vi "Set CSR Mode.vi"(8 "error in (no error)":errorcluster, 10 "Bandpass resolution (per grating line)":enum16{"3600", "1800", "900", "450"}(ring), 11 "VISA resource name":refnum<visa-resource-name>) -> (0 "error out":errorcluster, 2 "Bandpass Value":dbl[unit] min=0.0 max=0.016777215000000012 step=1.0000000000000007e-11 format="%.2f", 3 "VISA resource name out":refnum<visa-resource-name>)   [LabVIEW 2009, in "Digikrom DK24x.lvlib"]
doc: "This command sets monochromator to Constant Spectral Resolution mode. The slit width will vary throughout a scan. This is useful, for example, where measurement of a constant interval of frequency is desired (spectral power distribution measurements). See DK24x manual, appendix E, page 39.\n\nThe instrument can be removed from the CSR mode in the following five ways:\n1. By selecting a specific slit setting\n2. By selecting a new grating\n3. By resetting, recalibrating, or clearing the instrument\n4. By selecting the TEST function\n5. By removing power from the instrument\n\nGrating (lines/mm) Allowed Bandpass Values(nanometers)\n2400 1.50 0.75 0.37 0.18\n1200 3.00 1.50 0.75 0.37\n600 6.00 3.00 1.50 0.75\n300 12.0 6.00 3.00 1.50\n150 24.0 12.0 6.00 3.00\n75 48.0 24.0 12.0 6.00"
uses:
  Digikrom DK24x.lvlib
  Private/Command.ctl
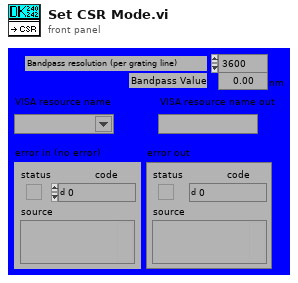
[diagram p1: front panel]
types:
  T1 = typedef "Digikrom DK24x.lvlib/Command.ctl" = u8
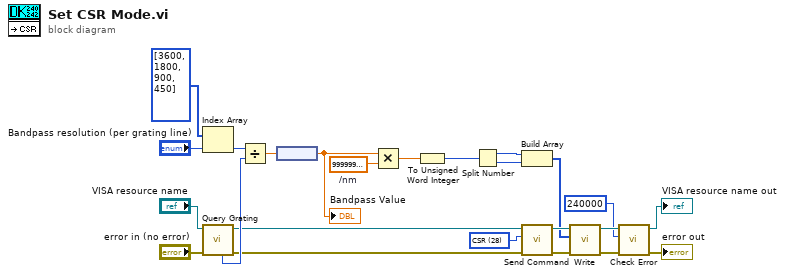
[diagram p0: block diagram]
diagram:
  w1 = T1 28 items=["Cancel"=24, "Clear"=25, "CSR"=28, "Echo"=27, "Filter"=15, "Gcal"=18, "Goto"=16, "Grtid?"=19, "Grtsel"=26, "NOVRAM Read"=56, "NOVRAM Write"=59, "Reset"=255, "Scan"=12, "Scan Up"=9, "Scan Down"=3, "Serial?"=33, "Slew Up"=8, "Slew Down"=2, "Slit Reset"=43, "Slit?"=30, "Sltadj"=14, "Speed"=13, "Sspeed?"=21, "Step Down"=1, "Step Up"=7, "S1adj"=31, "S2adj"=32, "S3adj"=34, "S1cal"=22, "S2cal"=23, "S3cal"=35, "Test"=17, "Type"=57, "Wave?"=29, "Zero"=52] ("Command")
  w22 = dbl[unit] 99999999999.99992  # /nm
  n1 = Index Array(array=u32[] [3600, 1800, 900, 450], index="Bandpass resolution (per grating line)") -> (element=w9:u32)
  n2 = call "Query Grating.vi"("error in (no error)"="error in (no error)", "VISA resource name"="VISA resource name") -> ("error out"=w3:errorcluster, "VISA resource name out"=w4:refnum<visa-resource-name>, "GR/MM"=w11:u16)  [unwired: 7 out]
  n3 = Divide(x=w9, y=w11) -> (x/y=w8:dbl)
  n4 = node(w8) -> (w2:dbl[unit])
  "Bandpass Value" <- w2
  n5 = Multiply(x=w2, y=w22) -> (x*y=w21:dbl)
  n6 = To Unsigned Word Integer(number=w21) -> (unsigned 16bit integer=w12:u16)
  n7 = Split Number(x=w12) -> (hi(x)=w24:u8, lo(x)=w23:u8)
  n8 = Build Array(w24, w23) -> (w13:u8[])
  n9 = call "Send Command.vi"("error in (no error)"=w3, "Command"=w1, "VISA resource name"=w4) -> ("error out"=w17:errorcluster, "VISA resource name out"=w16:refnum<visa-resource-name>)  [unwired: 7 out]
  n10 = call "Write.vi"("error in (no error)"=w17, "Byte Array"=w13, "VISA resource name"=w16) -> ("error out"=w20:errorcluster, "VISA resource name out"=w19:refnum<visa-resource-name>)  [unwired: 7 out]
  n11 = call "Check Error.vi"("error in"=w20, "timeout"=240000, "VISA resource name in"=w19) -> ("error out"=→"error out":errorcluster, "VISA resource name out"=→"VISA resource name out":refnum<visa-resource-name>)  [unwired: 7 out]
